vi "Agilent VNA Restore.vi"(7 "Agilent VNA":T1, 8 "error in (no error)":errorcluster, 11 "VISA Resource Name":refnum<visa-resource-name>) -> (0 "error out":errorcluster {"code" format="%.0x"}, 3 "dup VISA Resource Name":refnum<visa-resource-name>)   [LabVIEW 2011]
uses:
  TypeDefs/Agilent VNA Instrument Info.ctl
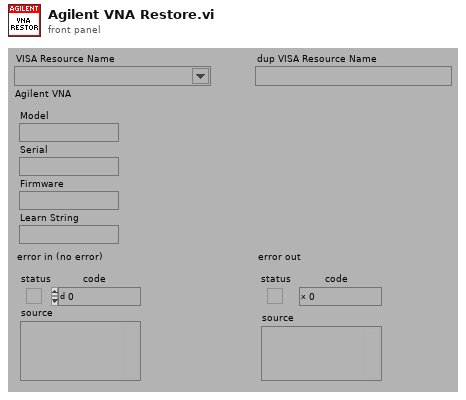
[diagram p1: front panel]
types:
  T1 = typedef "Agilent VNA Instrument Info.ctl" = cluster{"Model":string, "Serial":string, "Firmware":string, "Learn String":string}
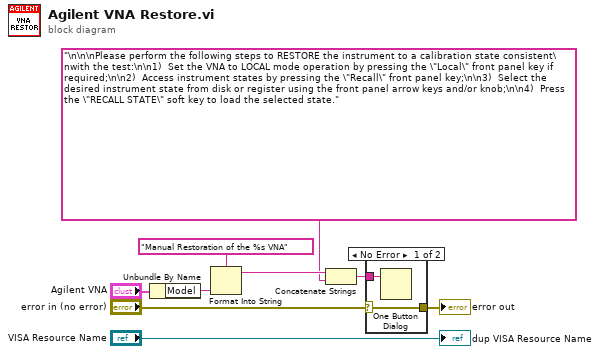
[diagram p0: block diagram]
diagram:
  n1 = Unbundle By Name("Agilent VNA") -> ("Model"=w7:string)
  n2 = Format Into String(format string="Manual Restoration of the %s VNA", w7) -> (resulting string=w6:string)  [unwired: 2 in, 1 out]
  n3 = Concatenate Strings(w6, "\n\n\nPlease perform the following steps to RESTORE the instrument to a calibration state consistent\nwith the test:\n\n1)  Set the VNA to LOCAL mode operation by pressing the \"Local\" front panel key if required;\n\n2)  Access instrument states by pressing the \"Recall\" front panel key;\n\n3)  Select the desired instrument state from disk or register using the front panel arrow keys and/or knob;\n\n4)  Press the \"RECALL STATE\" soft key to load the selected state.") -> (w4:string)
  n4 = case shown="No Error" "error in (no error)" {
    selector: "error in (no error)" -> [w10 w12]
    tunnel: w4 -> [w11 _]
    tunnel: [w10 w12] -> w2
    frame No Error {
      n5 = One Button Dialog(message=w11) -> ()  [unwired: 2 out]
    }
    frame Error {
    }
  }
  "error out" <- w2
  "dup VISA Resource Name" <- "VISA Resource Name"
